vi "SPC_get_scan_clk_state.vi"(8 "Error In":errorcluster, 10 "Module No":i16 min=0 max=7 step=1, 11 "DLL Path":path) -> (0 "Error Out":errorcluster, 2 "Module No":i16 min=0 max=7 step=1, 3 "DLL Path":path, 4 "Scanning Clocks\nstate value":i16, 5 "Clock Status":T1)   [LabVIEW 2017]
doc: "The procedure sets \"scan_state\" according to the actual state of the scanning clocks on the SPC module ‘mod_no’. \nScan_state value is valid only when the module’s measurement mode is set to ‘Scan In’ ( by setting parameter MODE using SPC_set_parameter procedure). Otherwise the procedure returns error code -SPC_BAD_FUNC. \nThe procedure works only for SPC-830/140/15x/930/160 modules and SPC-7x0 modules with FPGA version greater than 300(hex). For other modules it returns error code -SPC_BAD_FUNC (FPGA version can be checked using SPC_get_version procedure).\nScan_state bits should be interpreted as follows:\nBit mask value (hex): \n1 – External Pixel Clock present \n2 – Line Clock present\n4 – Frame Clock present\n\nThis VI interprets the bit mask as a boolean cluster.\n\ninfo@becker-hickl.com"
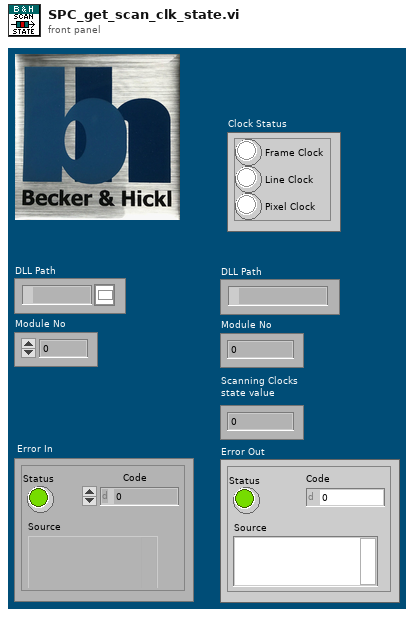
[diagram p1: front panel]
types:
  T1 = cluster{"Frame Clock":bool, "Line Clock":bool, "Pixel Clock":bool}
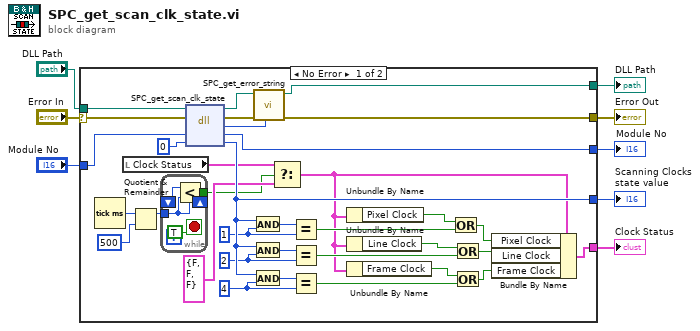
[diagram p0: block diagram]
diagram:
  n1 = case shown="No Error" "Error In" {
    selector: "Error In" -> [w34 w49]
    tunnel: "DLL Path" -> [w42 w48]
    tunnel: [w41 w49] -> w6
    tunnel: [w39 w48] -> w5
    tunnel: "Module No" -> [w37 w47]
    tunnel: [w36 w47] -> w3
    tunnel: [w35 _] -> w2
    tunnel: [w29 _] -> w1
    frame No Error {
      w24 = i16 4 ("y")
      w26 = i16 2 ("y")
      w28 = i16 1 ("y")
      n2 = Tick Count (ms)() -> (millisecond timer value=w13:u32)
      n3 = local read "Clock Status"() -> (w16:T1)
      n4 = Quotient & Remainder(x=w13, y=u32 500) -> (x-y*floor(x/y)=w10:u32)  [unwired: 1 out]
      n5 = while {
        tunnel: w10 -> [w43]
        shift-right: [w43] -> _
        shift-left: _ -> [w45]
        tunnel: [w44] -> w9
        stop <- TRUE stop-if-true
        n6 = Less?(x=w45, y=w43) -> (x < y?=w44:bool)
      }
      n7 = dll-call lib="D:/spcm/lib/lab_view/lv10.0/spcm32.dll" fn="SPC_get_scan_clk_state"(path in=w42, error in=w34, "mod_no"=w37, "scan_state"=i16 0 ("Scanning Clocks\nstate value")) -> (path out=w40:path, error out=w38:errorcluster, "return type"=w32:i16, "mod_no"=w36:i16, "scan_state"=w35:i16)  [unwired: 1 in]
      n8 = And(x=w35, y=w28) -> (x .and. y?=w27:i16)
      n9 = And(x=w35, y=w26) -> (x .and. y?=w25:i16)
      n10 = And(x=w35, y=w24) -> (x .and. y?=w23:i16)
      n11 = call "SPC_get_error_string.vi"("ErrorID"=w32, "Error In"=w38, "DLL Path"=w40) -> ("Error Out"=w41:errorcluster, "DLL Path"=w39:path)  [unwired: 6 in, 1 out]
      n12 = Select(t=w16, s=w9, f=T1 {"Frame Clock"=FALSE, "Line Clock"=FALSE, "Pixel Clock"=FALSE} ("Clock Status")) -> (s? t:f=w15:T1)
      n13 = Equal?(x=w27, y=w28) -> (x = y?=w33:bool)
      n14 = Equal?(x=w25, y=w26) -> (x = y?=w31:bool)
      n15 = Equal?(x=w23, y=w24) -> (x = y?=w30:bool)
      n16 = Unbundle By Name(w15) -> ("Pixel Clock"=w17:bool)
      n17 = Unbundle By Name(w15) -> ("Line Clock"=w19:bool)
      n18 = Unbundle By Name(w15) -> ("Frame Clock"=w21:bool)
      n19 = Or(x=w17, y=w33) -> (x .or. y?=w18:bool)
      n20 = Or(x=w19, y=w31) -> (x .or. y?=w20:bool)
      n21 = Or(x=w21, y=w30) -> (x .or. y?=w22:bool)
      n22 = Bundle By Name(cluster=w15, "Pixel Clock"=w18, "Line Clock"=w20, "Frame Clock"=w22) -> (w29:T1)
    }
    frame Error {
    }
  }
  "DLL Path" <- w5
  "Error Out" <- w6
  "Module No" <- w3
  "Scanning Clocks\nstate value" <- w2
  "Clock Status" <- w1
